vi "StressTester.vi"() -> ()   [LabVIEW 2013]
uses:
  Team Data.ctl
  <vilib>/httpClient/MultipartData.ctl
  <vilib>/xml/Close Reference(Node).vi
  <vilib>/httpClient/LabVIEWHTTPClient.lvlib
  <vilib>/xml/NI_XML.lvlib
  <resource>/objmgr/DOMUserDefRef.rc
panel:
  in  "Schedule Path (For Teams)":path=path "E:/Code/LabVIEW/FLL 2.1/schedule.csv"
  in  "Delay (ms)":u32
  in  "Entry Mode":enum16{"Automatic", "Manual"}(ring)
  in  "Elements Path (For Elements":path=path "E:/Code/LabVIEW/FLL 2.1/Web Pages/Data.xml"
  in  "Mode":T1(ring)=enum."Randomize Teams/Rounds"
  in  "Runs":i32=30
  in  "Round":u16=2
  in  "Team":u16=543
  in  "Elements":cluster{"Name":string, "Value":string}[](array[cluster])=[{"Name"="Supply_Truck_On_Yellow", "Value"="Yes"}, {"Name"="Evac_Sign_Upright", "Value"="Yes"}, {"Name"="Cargo_Plane", "Value"="Light Blue"}, {"Name"="Tree_Branch_Below_Wires", "Value"="No"}, {"Name"="All_Waves_On_Mat", "Value"="No"}, {"Name"="Ambulance_In_Yellow", "Value"="Yes"}, {"Name"="Runway_Clear", "Value"="Yes"}, {"Name"="Construction_Relocation", "Value"="No"}, {"Name"="Base_Isolation", "Value"="Yes"}, {"Name"="Code_Construction", "Value"="0"}, {"Name"="Obstacles", "Value"="Dark Green"}, {"Name"="Progress", "Value"="Default"}, {"Name"="Family", "Value"="None"}, {"Name"="Safety-_People_In_Red", "Value"="3"}, {"Name"="Safety-_People_In_Yellow", "Value"="1"}, {"Name"="Pets", "Value"="1"}, {"Name"="Water", "Value"="1"}, {"Name"="Supplies-_In_Red", "Value"="7"}, {"Name"="Supplies-_In_Yellow", "Value"="5"}, {"Name"="Safe_Place", "Value"="Yes"}, {"Name"="Penalties-_Outside_Light_Blue", "Value"="0"}, {"Name"="Penalties-_Inside_Light_Blue", "Value"="3"}]
  in  "URL":string="http://localhost:8001/Control/Process_POST"
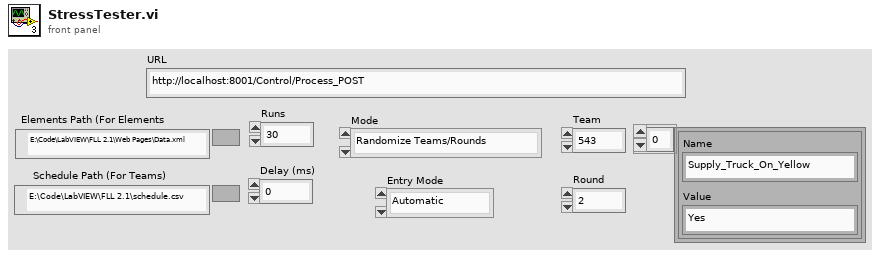
[diagram p1: front panel]
types:
  T1 = enum16{"Single Team/Round", "Randomize Teams/Rounds"}
  T2 = typedef "Team Data.ctl" = cluster{"Both":string, "Name":string, "GUID":u16, "Number":u16}
  T3 = typedef "LabVIEWHTTPClient.lvlib/MultipartData.ctl" = cluster{"Name":string, "Value":string, "File":path, "Filename":string, "MIME type":string}
  T4 = typedef "LabVIEWHTTPClient.lvlib/ClientHandle.ctl" = refnum<k1>
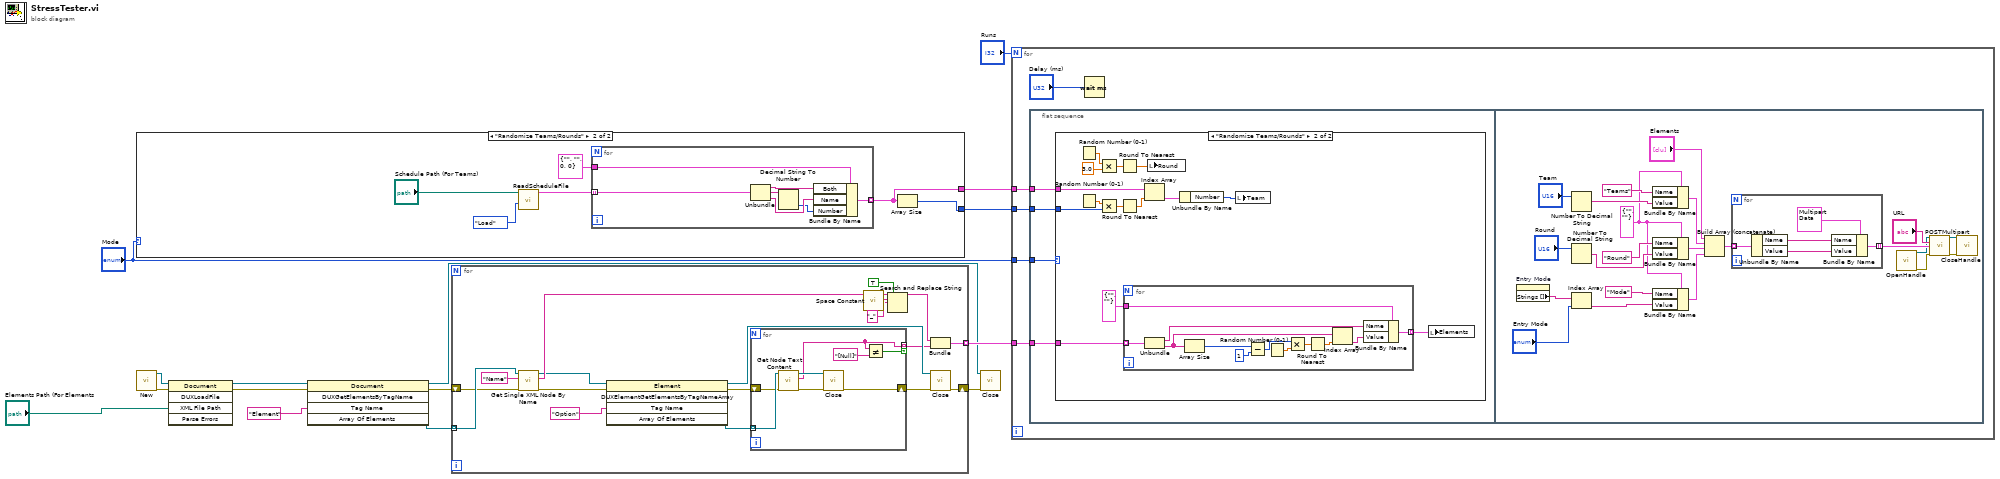
[diagram p0: block diagram]
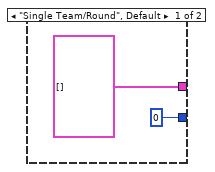
[diagram p2: hidden frame]
diagram:
  n1 = case shown="\"Randomize Teams/Rounds\"" "Mode" {
    tunnel: [T2[] [] ("Team Array Out") w18] -> w13
    tunnel: [0 w23] -> w12
    frame "Single Team/Round", Default {
    }
    frame "Randomize Teams/Rounds" {
      n2 = call "ReadScheduleFile.vi"("Enum"=enum16{"Load", "Get"}."Load", "Team Info / Schedule File"="Schedule Path (For Teams)") -> ("Team Information"=w20:cluster{string, "[0]":string, "[1]":string}[])  [unwired: 2 in, 7 out]
      n3 = for {
        tunnel: w20 -> [w30] mode=indexing
        tunnel: T2 {"Both"="", "Name"="", "GUID"=0, "Number"=0} ("Team Data") -> [w29]
        tunnel: [w28] -> w18 mode=indexing
        n4 = Unbundle(w30) -> (w27:string, "[0]"=w25:string, "[1]"=w26:string)
        n5 = Decimal String To Number(string=w25) -> (number=w24:i32)  [unwired: 2 in, 1 out]
        n6 = Bundle By Name(cluster=w29, "Both"=w27, "Name"=w26, "Number"=w24) -> (w28:T2)
      }
      n7 = Array Size(array=w18) -> (size(s)=w23:i32)
    }
  }
  n8 = call <vilib>:"New.vi"() -> ("error out"=w10:errorcluster, "DOM document out"=w11:refnum<k20>)  [unwired: 8 in]
  n9 = invoke class="Document" method="DUXLoadFile"(reference=w11, error in=w10, "XML File Path"="Elements Path (For Elements") -> (reference out=w8:refnum<k20>, error out=w7:errorcluster)  [unwired: 2 in, 3 out]
  n10 = invoke class="Document" method="DUXGetElementsByTagName"(reference=w8, error in=w7, "Tag Name"="Element") -> (reference out=w1:refnum<k20>, error out=w4:errorcluster, "Array Of Elements"=w5:refnum<k20>[])  [unwired: 2 in, 2 out]
  n11 = for {
    tunnel: w5 -> [w48] mode=indexing
    shift-right: [w41] -> w2
    shift-left: w4 -> [w47]
    tunnel: [w33] -> w3 mode=indexing
    n12 = call "Get Single XML Node By Name.vi"("error in (no error)"=w47, "Tag Name"="Name", "Parent Element"=w48) -> ("error out"=w38:errorcluster, "node text"=w45:string, "Parent Element Out"=w40:refnum<k20>)  [unwired: 6 in]
    n13 = invoke class="Element" method="DUXElementGetElementsByTagNameArray"(reference=w40, error in=w38, "Tag Name"="Option") -> (reference out=w39:refnum<k20>, error out=w35:errorcluster, "Array Of Elements"=w36:refnum<k20>[])  [unwired: 2 in, 2 out]
    n14 = for {
      tunnel: w36 -> [w56] mode=indexing
      shift-right: [w53] -> w34
      shift-left: w35 -> [w55]
      tunnel: [w51] -> w31 mode=indexing if=w49
      n15 = call <vilib>:"Get Node Text Content.vi"("error in (no error)"=w55, "node in"=w56) -> ("error out"=w54:errorcluster, "node text"=w51:string, "node out"=w52:refnum<k20>)  [unwired: 7 in]
      n16 = call-poly <vilib>:"Close.vi"("error in (no error)"=w54, "node"=w52) -> ("error out"=w53:errorcluster)  [unwired: 7 in]
      n17 = Not Equal?(x=w51, y="[Null]") -> (x != y?=w49:bool)
    }
    n18 = call <vilib>:"Space Constant.vi"() -> ("String"=w44:string)
    n19 = Search and Replace String(replace all?=TRUE ("replace all? (F)"), input string=w45, search string=w44, replace string="_" ("replace string (\"\")")) -> (result string=w32:string)  [unwired: 4 in, 3 out]
    n20 = Bundle("result string"=w32, w31) -> (w33:cluster{"result string":string, string[]})  [unwired: 1 in]
    n21 = call-poly <vilib>:"Close.vi"("error in (no error)"=w34, "node"=w39) -> ("error out"=w41:errorcluster)  [unwired: 7 in]
  }
  n22 = call-poly <vilib>:"Close.vi"("error in (no error)"=w2, "node"=w1) -> ()  [unwired: 7 in, 1 out]
  n23 = for {
    N: "Runs" -> [_]
    tunnel: "Mode" -> [w58]
    tunnel: w13 -> [w61]
    tunnel: w12 -> [w60]
    tunnel: w3 -> [w59]
    n24 = flat-sequence {
      tunnel: w61 -> [w65]
      tunnel: w60 -> [w64]
      tunnel: w59 -> [w63]
      tunnel: w58 -> [w62]
      frame #0 {
        n25 = case shown="\"Randomize Teams/Rounds\"" w62 {
          tunnel: w65 -> [_ w76]
          tunnel: w64 -> [_ w78]
          tunnel: w63 -> [_ w68]
          frame "Single Team/Round", Default {
          }
          frame "Randomize Teams/Rounds" {
            n26 = Random Number (0-1)() -> (number: 0 to 1=w72:dbl)
            n27 = Random Number (0-1)() -> (number: 0 to 1=w79:dbl)
            n28 = Multiply(x=w72, y=3.0) -> (x*y=w70:dbl)
            n29 = Multiply(x=w79, y=w78) -> (x*y=w77:dbl)
            n30 = Round To Nearest(number=w70) -> (nearest integer value=w69:dbl)
            n31 = Round To Nearest(number=w77) -> (nearest integer value=w75:dbl)
            n32 = for {
              tunnel: w68 -> [w83] mode=indexing
              tunnel: cluster{"Name":string, "Value":string} {"Name"="", "Value"=""} ("Scoring Element") -> [w91]
              tunnel: [w90] -> w66 mode=indexing
              n33 = Unbundle(w83) -> ("result string"=w82:string, w81:string[])
              n34 = Array Size(array=w81) -> (size(s)=w87:i32)
              n35 = Subtract(x=w87, y=1) -> (x-y=w85:i32)
              n36 = Random Number (0-1)() -> (number: 0 to 1=w88:dbl)
              n37 = Multiply(x=w85, y=w88) -> (x*y=w80:dbl)
              n38 = Round To Nearest(number=w80) -> (nearest integer value=w84:dbl)
              n39 = Index Array(array=w81, index=w84) -> (element=w89:string)
              n40 = Bundle By Name(cluster=w91, "Name"=w82, "Value"=w89) -> (w90:cluster{"Name":string, "Value":string})
            }
            n41 = Index Array(array=w76, index=w75) -> (element=w74:T2)
            n42 = local write "Round"(w69) -> ()
            n43 = Unbundle By Name(w74) -> ("Number"=w73:u16)
            n44 = local write "Team"(w73) -> ()
            n45 = local write "Elements"(w66) -> ()
          }
        }
      }
      frame #1 {
        w97 = cluster{"Name":string, "Value":string} {"Name"="", "Value"=""} ("Scoring Element")
        n46 = property on="Entry Mode" class="Enum (strict)"() -> ("Strings []"=w95:string[])  [unwired: 2 in, 2 out]
        n47 = Number To Decimal String(number="Team") -> (decimal integer string=w107:string)  [unwired: 1 in]
        n48 = Number To Decimal String(number="Round") -> (decimal integer string=w111:string)  [unwired: 1 in]
        n49 = Index Array(array=w95, index="Entry Mode") -> (element=w93:string)
        n50 = Bundle By Name(cluster=w97, "Name"="Teams", "Value"=w107) -> (w109:cluster{"Name":string, "Value":string})
        n51 = Bundle By Name(cluster=w97, "Name"="Round", "Value"=w111) -> (w113:cluster{"Name":string, "Value":string})
        n52 = Bundle By Name(cluster=w97, "Name"="Mode", "Value"=w93) -> (w92:cluster{"Name":string, "Value":string})
        n53 = Build Array (concatenate)("Elements", w109, w113, w92) -> (w105:cluster{"Name":string, "Value":string}[])
        n54 = for {
          tunnel: w105 -> [w118] mode=indexing
          tunnel: [w114] -> w103 mode=indexing
          n55 = Unbundle By Name(w118) -> ("Name"=w116:string, "Value"=w115:string)
          n56 = Bundle By Name(cluster=T3 {"Name"="", "Value"="", "File"=path "", "Filename"="", "MIME type"="application/octet-stream"} ("Element"), "Name"=w116, "Value"=w115) -> (w114:T3)
        }
        n57 = call <vilib>:"OpenHandle.vi"() -> ("client handle out"=w101:T4, "error out"=w100:errorcluster)  [unwired: 14 in]
        n58 = call <vilib>:"POSTMultipart.vi"("client handle"=w101, "url"="URL", "data"=w103, "error in (no error)"=w100) -> ("client handle out"=w98:T4, "error out"=w99:errorcluster)  [unwired: 8 in, 2 out]
        n59 = call <vilib>:"CloseHandle.vi"("client handle"=w98, "error in (no error)"=w99) -> ()  [unwired: 13 in, 1 out]
      }
    }
    n60 = Wait (ms)(milliseconds to wait="Delay (ms)") -> ()  [unwired: 1 out]
  }
